vi "heartbeat.vi"(0 "object in":refnum<class "212format_work.lvclass">, 1 "in":T1, 5 "error in (no error)":errorcluster) -> (14 "object out":refnum<class "212format_work.lvclass">, 15 "out":T2, 19 "error out":errorcluster)   [LabVIEW 2016, in "212format_work.lvclass"]
uses:
  212format_work.lvclass
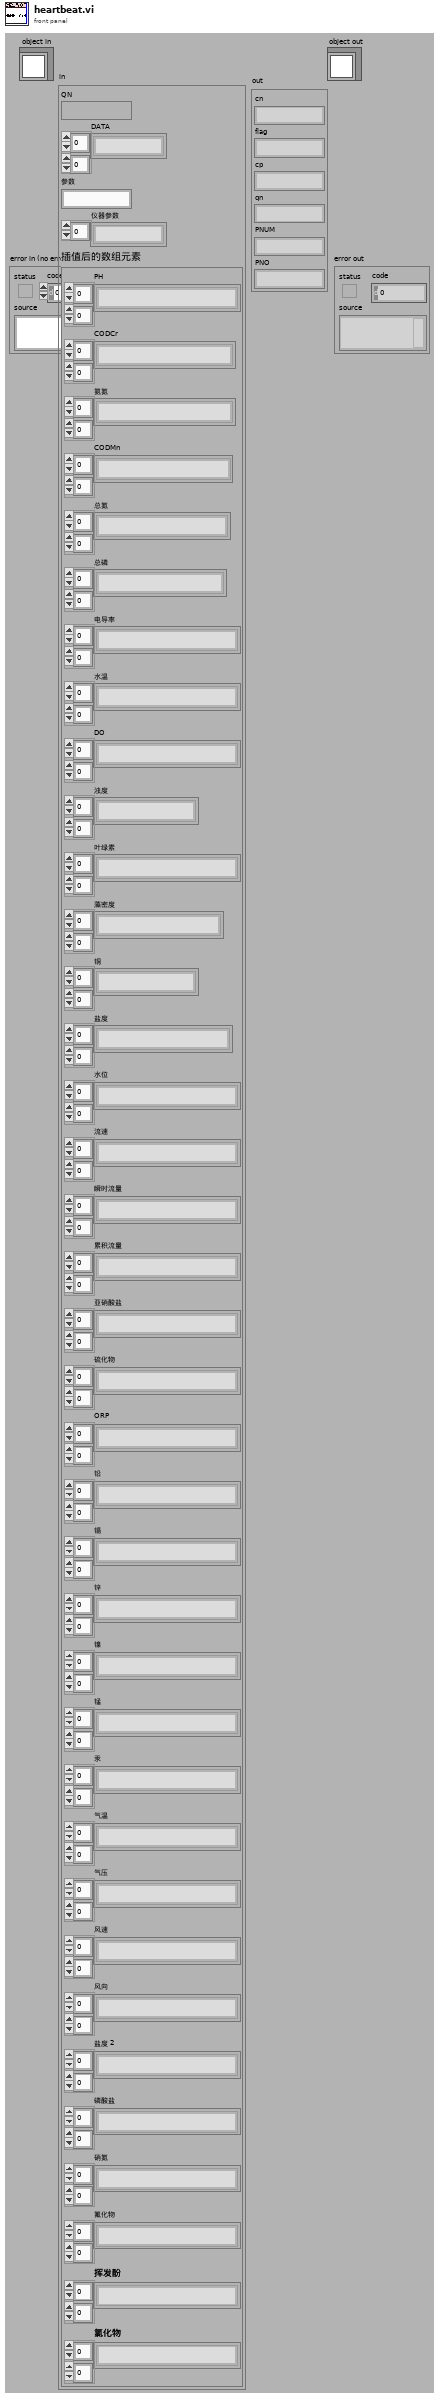
[diagram p1: front panel]
types:
  T1 = cluster{"QN":string, "DATA":string[][], "参数":string, "仪器参数":string[], "插值后的数组元素":cluster{"PH":string[][], "CODCr":string[][], "氨氮":string[][], "CODMn":string[][], "总氮":string[][], "总磷":string[][], "电导率":string[][], "水温":string[][], "DO":string[][], "浊度":string[][], "叶绿素":string[][], "藻密度":string[][], "铜":string[][], "盐度":string[][], "水位":string[][], "流速":string[][], "瞬时流量":string[][], "累积流量":string[][], "亚硝酸盐":string[][], "硫化物":string[][], "ORP":string[][], "铅":string[][], "镉":string[][], "锌":string[][], "镍":string[][], "锰":string[][], "汞":string[][], "气温":string[][], "气压":string[][], "风速":string[][], "风向":string[][], "盐度 2":string[][], "磷酸盐":string[][], "硝氮":string[][], "氟化物":string[][], "挥发酚":string[][], "氯化物":string[][]}}
  T2 = cluster{"cn":string, "flag":string, "cp":string, "qn":string, "PNUM":string, "PNO":string}
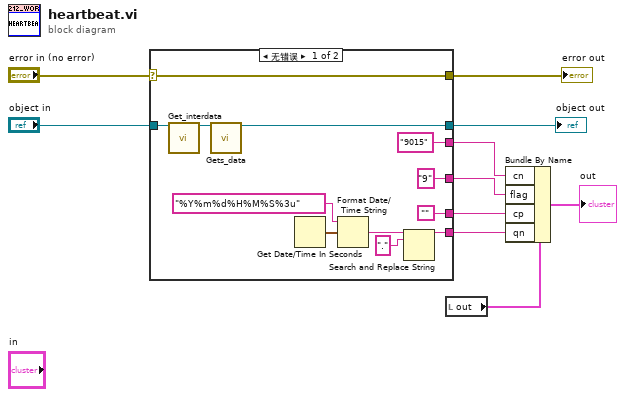
[diagram p0: block diagram]
diagram:
  n1 = case shown="无错误" "error in (no error)" {
    selector: "error in (no error)" -> [w22 w24]
    tunnel: [w22 w24] -> w9
    tunnel: [w18 w23] -> w7
    tunnel: "object in" -> [w20 w23]
    tunnel: ["" _] -> w2
    tunnel: ["9015" ("ST") _] -> w4
    tunnel: ["9" ("ST") _] -> w3
    tunnel: [w11 _] -> w1
    frame No Error {
      n2 = call-dynamic "Get_interdata.vi"("object in"=w20) -> ("object out"=w19:refnum<class "212format_work.lvclass">)  [unwired: 16 in, 2 out]
      n3 = call-dynamic "Gets_data.vi"("object in"=w19) -> ("object out"=w18:refnum<class "212format_work.lvclass">)  [unwired: 16 in, 2 out]
      n4 = Get Date/Time In Seconds() -> (seconds since 1Jan1904=w14:timestamp)
      n5 = Format Date/Time String(time format string (%c)="%Y%m%d%H%M%S%3u" ("时间格式字符串(%c)"), seconds (now)=w14) -> (date/time string=w13:string)  [unwired: 1 in]
      n6 = Search and Replace String(input string=w13, search string="." ("搜索字符串")) -> (result string=w11:string)  [unwired: 6 in, 3 out]
    }
    frame Error {
    }
  }
  "error out" <- w9
  "object out" <- w7
  n7 = local read "out"() -> (w6:T2)
  n8 = Bundle By Name(cluster=w6, "cn"=w4, "flag"=w3, "cp"=w2, "qn"=w1) -> (→"out":T2)
